vi "get_instance.vi"(8 "error in (no error)":errorcluster, 11 "singleton in":refnum<class "singleton.lvclass">) -> (0 "error out":errorcluster, 3 "instance handle":T1)   [LabVIEW 2020, in "singleton.lvclass"]
uses:
  singleton.lvclass
  Typedefs/Instance Handle.ctl
  singleton.lvclass/singleton.ctl
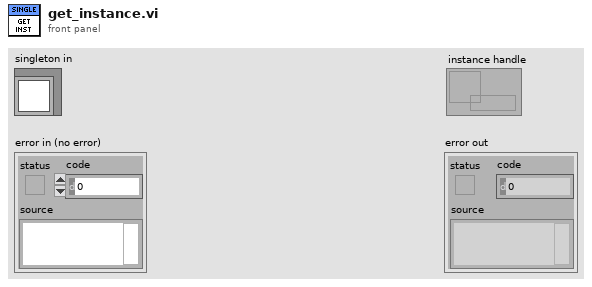
[diagram p1: front panel]
types:
  T1 = typedef "singleton.lvclass/Instance Handle.ctl" = refnum<data-value>
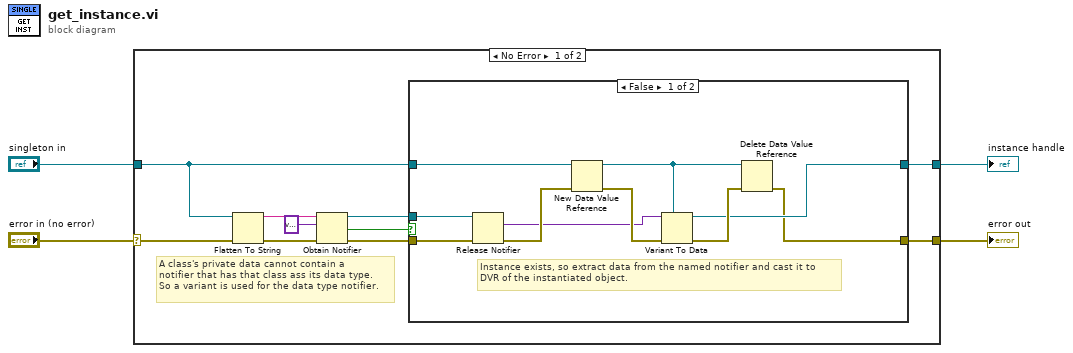
[diagram p0: block diagram]
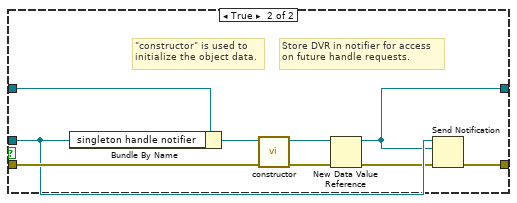
[diagram p2: hidden frame]
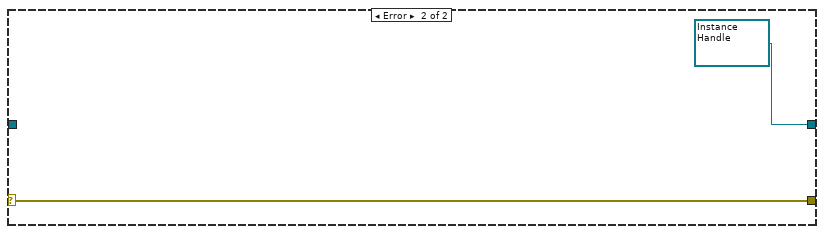
[diagram p3: hidden frame]
diagram:
  n1 = case shown="No Error" "error in (no error)" {
    selector: "error in (no error)" -> [w14 w35]
    tunnel: [w7 w35] -> w3
    tunnel: "singleton in" -> [w10 _]
    tunnel: [w6 T1 refnum ("data value reference")] -> w1
    frame No Error {
      # "A class's private data cannot contain a\nnotifier that has that class ass its data type.\nSo a variant is used for the data type notifier."
      n2 = Flatten To String(anything=w10, error in (no error)=w14) -> (data string=w12:string, error out=w13:errorcluster)  [unwired: 2 in, 1 out]
      n3 = Obtain Notifier(name (unnamed)=w12, notification data type=variant ("element data type"), error in (no error)=w13) -> (notifier out=w8:refnum<notifier>, created new?=w5:bool, error out=w9:errorcluster)  [unwired: 1 in]
      n4 = case shown="False" w5 {
        tunnel: w10 -> [w21 w33]
        tunnel: w9 -> [w24 w31]
        tunnel: w8 -> [w23 w29]
        tunnel: [w15 w26] -> w7
        tunnel: [w16 w25] -> w6
        frame False {
          # "Instance exists, so extract data from the named notifier and cast it to\nDVR of the instantiated object."
          n5 = Release Notifier(notifier=w23, error in (no error)=w24) -> (last notification=w19:variant, error out=w22:errorcluster)  [unwired: 1 in, 1 out]
          n6 = New Data Value Reference(data value=w21, error in=w22) -> (data value reference=w17:refnum<data-value>, error out=w20:errorcluster)
          n7 = Variant To Data(error in=w20, type=w17, Variant=w19) -> (data=w16:refnum<data-value>, error out=w18:errorcluster)
          n8 = Delete Data Value Reference(data value reference=w17, error in=w18) -> (error out=w15:errorcluster)  [unwired: 1 out]
        }
        frame True {
          # "Store DVR in notifier for access\non future handle requests."
          # "\"constructor\" is used to\ninitialize the object data."
          n9 = Bundle By Name(cluster=w33, "singleton handle notifier"=w29) -> (w32:refnum<class "singleton.lvclass">)
          n10 = call-dynamic "constructor.vi"("error in (no error)"=w31, "singleton in"=w32) -> ("error out"=w27:errorcluster, "singleton out"=w30:refnum<class "singleton.lvclass">)  [unwired: 8 in]
          n11 = New Data Value Reference(data value=w30, error in=w27) -> (data value reference=w25:refnum<data-value>, error out=w28:errorcluster)
          n12 = Send Notification(notification=w25, notifier=w29, error in (no error)=w28) -> (error out=w26:errorcluster)  [unwired: 1 out]
        }
      }
    }
    frame Error {
    }
  }
  "error out" <- w3
  "instance handle" <- w1
